vi "Bird (SubVI).vi"(6 "a":dbl=-0.15, 8 "Jump":bool, 9 "Reset":bool, 10 "Jump speed":dbl=2.0, 11 "Ini Position":dbl=50.0 format="%#_13g") -> (3 "Position":dbl format="%.2f")   [LabVIEW 2013]
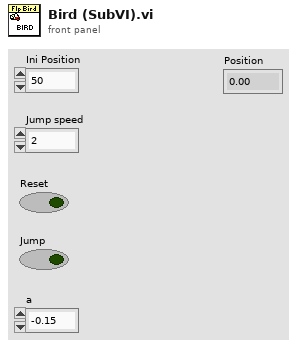
[diagram p1: front panel]
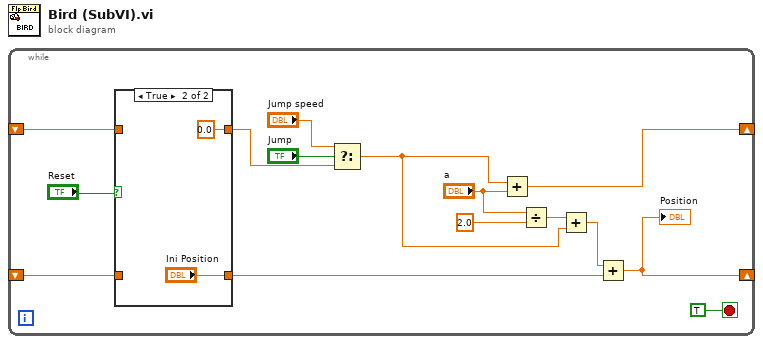
[diagram p0: block diagram]
diagram:
  n1 = while {
    shift-right: [w14] -> _
    shift-left: _ -> [w4]
    shift-right: [w9] -> _
    shift-left: _ -> [w3]
    stop <- TRUE stop-if-true
    n2 = case shown="True" "Reset" {
      tunnel: [w17 0.0] -> w5
      tunnel: w4 -> [w17 _]
      tunnel: w3 -> [w16 _]
      tunnel: [w16 "Ini Position"] -> w2
      frame False {
      }
      frame True {
      }
    }
    n3 = Select(t="Jump speed", s="Jump", f=w5) -> (s? t:f=w7:dbl)
    n4 = Add(x=w7, y="a") -> (x+y=w14:dbl)
    n5 = Divide(x="a", y=2.0) -> (x/y=w11:dbl)
    n6 = Add(x=w11, y=w7) -> (x+y=w10:dbl)
    n7 = Add(x=w10, y=w2) -> (x+y=w9:dbl)
    "Position" <- w9
  }
